vi "Live imaging window queue handler.vi"(8 "error in (no error)":errorcluster, 9 "Sim":bool, 10 "timeout in ms":i32, 11 "Queue in":T1) -> (1 "timed out?":bool, 2 "Frame rate (Hz)":dbl format="Acquisition frame rate: %.1f fps", 3 "Element to queue":T2)   [LabVIEW 2013]
uses:
  Live graphs queue/Typedefs/Live imaging queue element.ctl
  <vilib>/vision/Image Controls.llb/IMAQ Image.ctl
  Typedefs/Live graph data queue ref.ctl
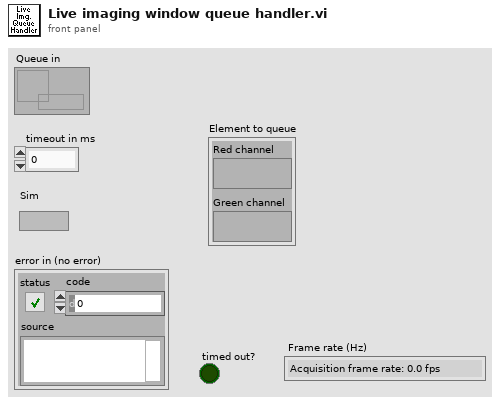
[diagram p1: front panel]
types:
  T1 = typedef "Live graph data queue ref.ctl" = refnum<queue>
  T2 = typedef "Live imaging queue element.ctl" = cluster{"Red channel":T3, "Green channel":T3}
  T3 = typedef "IMAQ Image.ctl" = refnum<image>
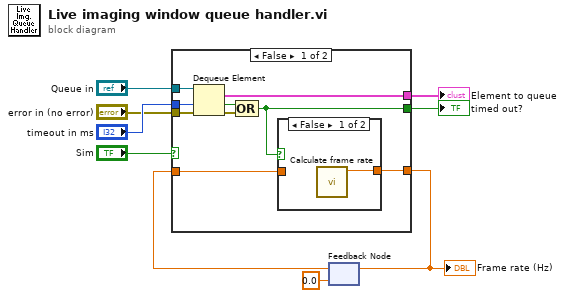
[diagram p0: block diagram]
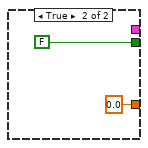
[diagram p3: hidden frame]
diagram:
  n1 = feedback #1(0.0 ("Frame rate (fps)")) -> (w1:dbl)
  n2 = case shown="False" "Sim" {
    tunnel: [w18 _] -> w6
    tunnel: "Queue in" -> [w17 _]
    tunnel: "error in (no error)" -> [w16 _]
    tunnel: "timeout in ms" -> [w15 _]
    tunnel: [w12 FALSE ("timed out?")] -> w7
    tunnel: [w11 0.0 ("Frame rate (fps)")] -> w2
    tunnel: w1 -> [w10 _]
    frame False {
      n3 = Dequeue Element(queue=w17, timeout in ms (-1)=w15, error in (no error)=w16) -> (element=w18:T2, timed out?=w13:bool, error out=w14:errorcluster)  [unwired: 1 out]
      n4 = Compound Arithmetic op=OR(w13, w14) -> (w12:bool)
      n5 = case shown="False" w12 {
        tunnel: [w19 w20] -> w11
        tunnel: w10 -> [_ w20]
        frame False {
          n6 = call "Calculate frame rate.vi"() -> ("Frame rate (fps)"=w19:dbl)  [unwired: 11 in]
        }
        frame True {
        }
      }
    }
    frame True {
    }
  }
  "timed out?" <- w7
  "Element to queue" <- w6
  "Frame rate (Hz)" <- w2
  n7 = feedback-in #1(w2) -> ()
